vi "Add Heartbeat.vi"(6 "Timeout":u16 format="%d ms", 8 "error in":errorcluster, 9 "Period":u16 format="%d ms", 10 "Node-ID":u8, 11 "CANopen Master in":refnum<class "CANopen Master.lvclass">) -> (0 "error out":errorcluster, 3 "CANopen Master out":refnum<class "CANopen Master.lvclass">)   [LabVIEW 2024, in "CANopen Master.lvlib" / "CANopen Master.lvclass"]
uses:
  CANopen Master.lvclass
  CANopen Master.lvclass/CANopen Master.ctl
  Heartbeat/Heartbeat.lvclass
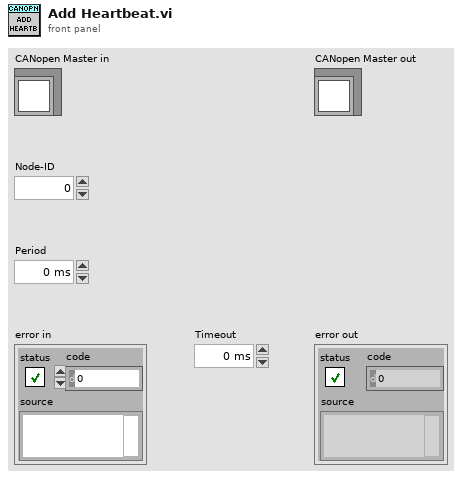
[diagram p1: front panel]
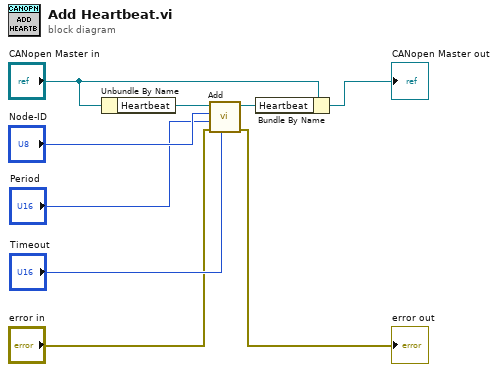
[diagram p0: block diagram]
diagram:
  n1 = Unbundle By Name("CANopen Master in") -> ("Heartbeat"=w7:refnum<class "Heartbeat.lvclass">)
  n2 = call "Add.vi"("Timeout"="Timeout", "error in"="error in", "Period"="Period", "Node-ID"="Node-ID", "Heartbeat in"=w7) -> ("error out"=→"error out":errorcluster, "Heartbeat out"=w2:refnum<class "Heartbeat.lvclass">)  [unwired: 5 in]
  n3 = Bundle By Name(cluster="CANopen Master in", "Heartbeat"=w2) -> (→"CANopen Master out":refnum<class "CANopen Master.lvclass">)
